vi "FLiNaK Viscosity.vi"(11 "Temperature (K)":dbl) -> (3 "FLiNaK Viscosity (Pa-s)":dbl)   [LabVIEW 2019]
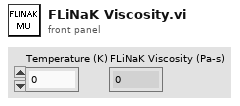
[diagram p1: front panel]
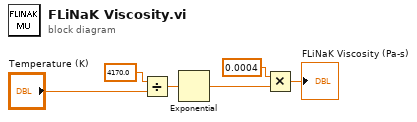
[diagram p0: block diagram]
diagram:
  n1 = Divide(x=4170.0 ("y"), y="Temperature (K)") -> (x/y=w3:dbl)
  n2 = Exponential(1:w3) -> (0:w4:dbl)
  n3 = Multiply(x=0.0004, y=w4) -> (x*y=→"FLiNaK Viscosity (Pa-s)":dbl)
